vi "VirtualMain.vi"() -> ()   [LabVIEW 2013, in "VirtualRobot.lvlib"]
uses:
  VirtualRobot.lvlib
panel:
  in  "Teleop Delay":u32=50
  in  "stop":bool
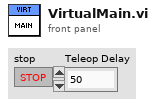
[diagram p1: front panel]
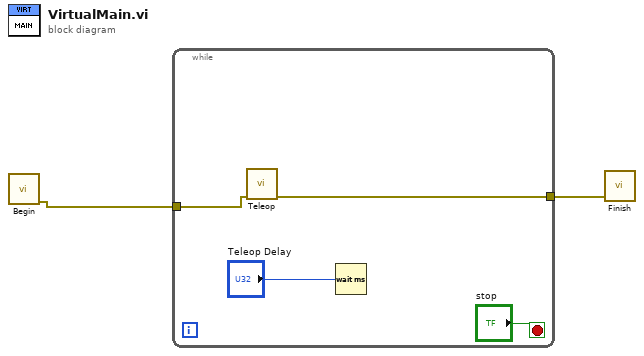
[diagram p0: block diagram]
diagram:
  n1 = call "Begin.vi"() -> ("error out"=w2:errorcluster)  [unwired: 11 in]
  n2 = while {
    tunnel: w2 -> [w4]
    tunnel: [w3] -> w1
    stop <- "stop" stop-if-true
    n3 = call "Teleop.vi"("error in (no error)"=w4) -> ("error out"=w3:errorcluster)  [unwired: 10 in]
    n4 = Wait (ms)(milliseconds to wait="Teleop Delay") -> ()  [unwired: 1 out]
  }
  n5 = call "Finish.vi"("error in (no error)"=w1) -> ()  [unwired: 11 in]
